vi "setUp.vi"(8 "error in (no error)":errorcluster, 11 "Test Runner.Project in":refnum<class "Test Runner.Project.lvclass">) -> (0 "error out":errorcluster, 3 "Test Runner.Project out":refnum<class "Test Runner.Project.lvclass">)   [LabVIEW 2013, in "Caraya.lvlib" / "Test Runner.Project.lvclass"]
uses:
  Test Runner.Project.lvclass
  Test Runner/Test Runner.lvclass
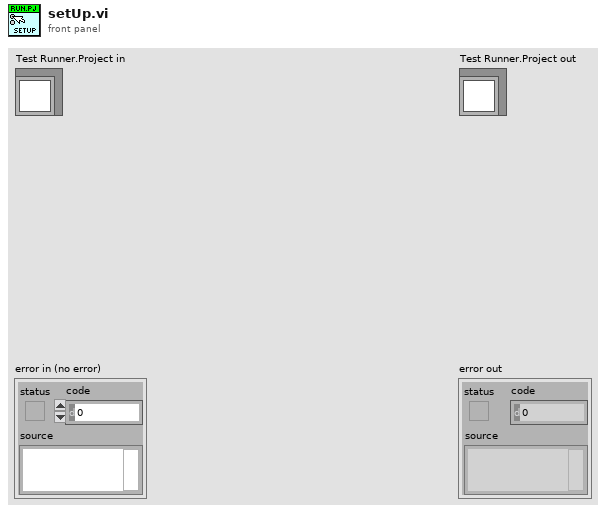
[diagram p1: front panel]
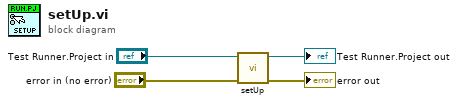
[diagram p0: block diagram]
diagram:
  n1 = call-parent "setUp.vi"("error in (no error)"="error in (no error)", "Test Runner in"="Test Runner.Project in") -> ("error out"=→"error out":errorcluster, "Test Runner out"=→"Test Runner.Project out":refnum<class "Test Runner.Project.lvclass">)  [unwired: 8 in]
